vi "csvHeaderGen.vi"() -> (2 "Valid Data in Buffer":i32, 3 "Data Buffer":string)   [LabVIEW 2019]
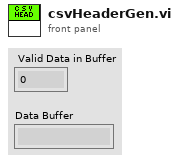
[diagram p1: front panel]
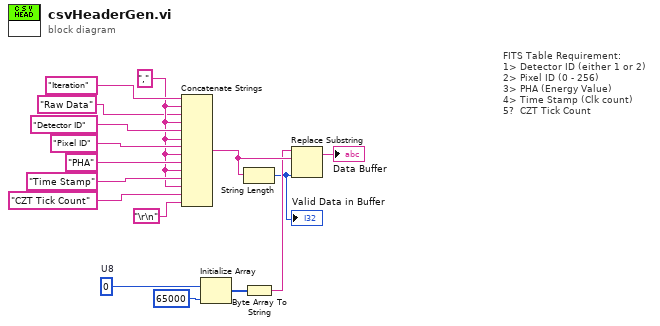
[diagram p0: block diagram]
diagram:
  w11 = u8 0  # U8
  w2 = "," (",")
  # "FITS Table Requirement:\n1> Detector ID (either 1 or 2)\n2> Pixel ID (0 - 256)\n3> PHA (Energy Value)\n4> Time Stamp (Clk count)\n5?  CZT Tick Count"
  n1 = Concatenate Strings("Iteration", w2, "Raw Data", w2, "Detector ID", w2, "Pixel ID", w2, "PHA", w2, "Time Stamp", w2, "CZT Tick Count", "\r\n" ("Row separator")) -> (w16:string)
  n2 = Initialize Array(w11, 65000 ("buffer size (bytes)")) -> (w12:u8[])
  n3 = String Length(string=w16) -> (length=w9:i32)
  "Valid Data in Buffer" <- w9
  n4 = Byte Array To String(unsigned byte array=w12) -> (string=w14:string)
  n5 = Replace Substring(2:w9, 4:w16, 5:w14) -> (1:→"Data Buffer":string)  [unwired: 1 in, 1 out]
